vi "Data entry form.vi"(8 "error in (no error)":errorcluster, 9 "Module?":bool, 10 "Position":dbl, 11 "Stack in":refnum<class "Stack.lvclass">) -> (0 "error out":errorcluster, 3 "Stack out":refnum<class "Stack.lvclass">)   [LabVIEW 2021, in "Stack.lvclass"]
uses:
  Stack.lvclass
  Stack.lvclass/Stack.ctl
panel:
  out "Date":string
  in  "Glue Batch":string
  in  "Operator":string
  in  "Component Tray ID":string
  in  "Assembly Tray ID":string
  in  "PUT ID":string
  in  "Baselayer ID":string
  in  "Toplayer ID":string
  in  "Submit":bool
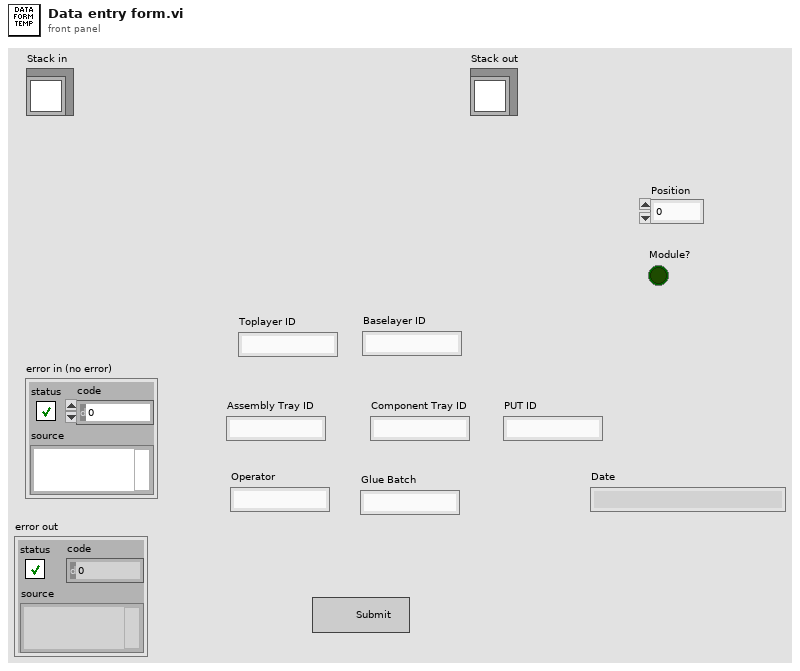
[diagram p1: front panel]
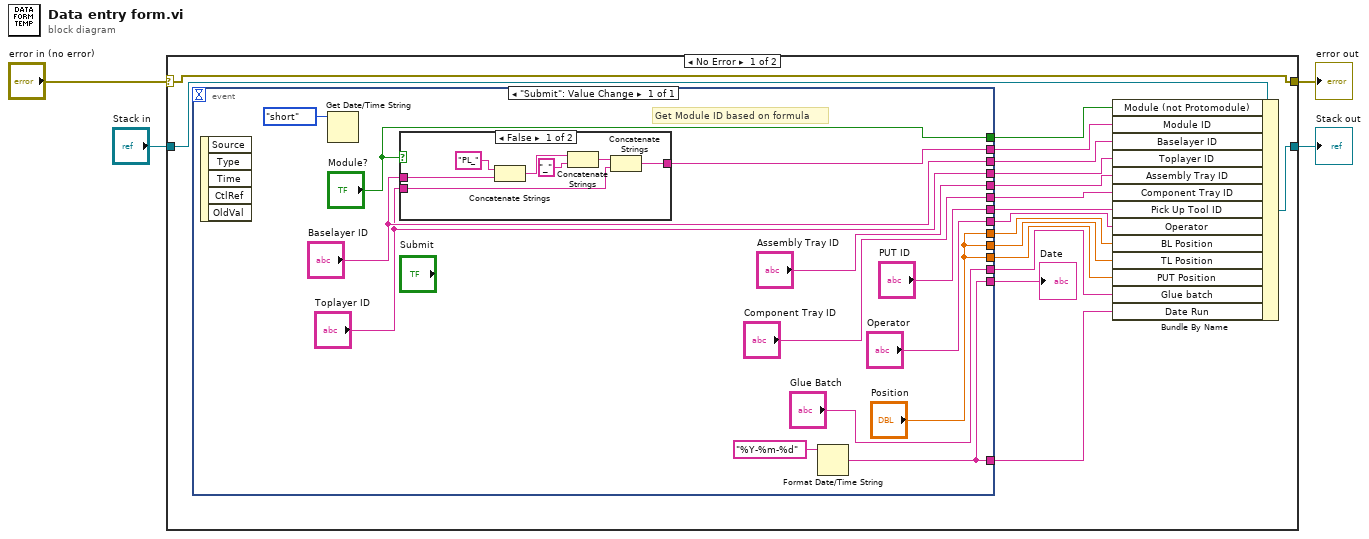
[diagram p0: block diagram]
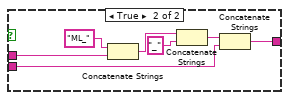
[diagram p2: hidden frame]
diagram:
  n1 = case shown="No Error" "error in (no error)" {
    selector: "error in (no error)" -> [w21 w50]
    tunnel: [w21 w50] -> w3
    tunnel: [w20 w49] -> w1
    tunnel: "Stack in" -> [w19 w49]
    frame No Error {
      n2 = event shown="[0] \"Submit\": Value Change" {
        selector: _ -> [_]
        dyn-events: _ -> [_]
        timeout: _ -> [_]
        tunnel: ["Toplayer ID"] -> w18
        tunnel: ["Baselayer ID"] -> w17
        tunnel: ["Component Tray ID"] -> w16
        tunnel: ["Assembly Tray ID"] -> w15
        tunnel: ["PUT ID"] -> w14
        tunnel: ["Operator"] -> w13
        tunnel: ["Module?"] -> w12
        tunnel: ["Position"] -> w11
        tunnel: ["Position"] -> w10
        tunnel: ["Position"] -> w9
        tunnel: [w27] -> w8
        tunnel: ["Glue Batch"] -> w7
        tunnel: [w22] -> w6
        tunnel: [w22] -> w5
        event "Submit": Value Change {
          # "Get Module ID based on formula"
          n3 = event-data() -> ()  [unwired: 1 in, 5 out]
          n4 = Get Date/Time String(date format (0)=enum16{"short", "long", "abbreviated"}."short") -> ()  [unwired: 2 in, 2 out]
          n5 = case shown="False" "Module?" {
            tunnel: "Baselayer ID" -> [w37 w44]
            tunnel: "Toplayer ID" -> [w36 w46]
            tunnel: [w35 w45] -> w27
            frame False {
              n6 = Concatenate Strings("PL_" ("string"), w37) -> (w41:string)
              n7 = Concatenate Strings(w41, "_" ("string")) -> (w40:string)
              n8 = Concatenate Strings(w40, w36) -> (w35:string)
            }
            frame True {
              n9 = Concatenate Strings("ML_" ("string"), w44) -> (w43:string)
              n10 = Concatenate Strings(w43, "_" ("string")) -> (w47:string)
              n11 = Concatenate Strings(w47, w46) -> (w45:string)
            }
          }
          n12 = Format Date/Time String(time format string (%c)="%Y-%m-%d") -> (date/time string=w22:string)  [unwired: 2 in]
        }
      }
      "Date" <- w5
      n13 = Bundle By Name(cluster=w19, "Module (not Protomodule)"=w12, "Module ID"=w8, "Baselayer ID"=w17, "Toplayer ID"=w18, "Assembly Tray ID"=w15, "Component Tray ID"=w16, "Pick Up Tool ID"=w14, "Operator"=w13, "BL Position"=w11, "TL Position"=w10, "PUT Position"=w9, "Glue batch"=w7, "Date Run"=w6) -> (w20:refnum<class "Stack.lvclass">)
    }
    frame Error {
    }
  }
  "error out" <- w3
  "Stack out" <- w1
